vi "sine_plotter.vi"() -> ()   [LabVIEW 2014]
panel:
  out "XY Graph":cluster{"XArray":dbl[], "YArray":dbl[]}(graph)
  out "YArray":dbl[](array[numeric])
  out "XArray":dbl[](array[numeric])
  out "XSteps":dbl
  in  "XEnd":dbl
  in  "XRes":dbl
  in  "XStart":dbl
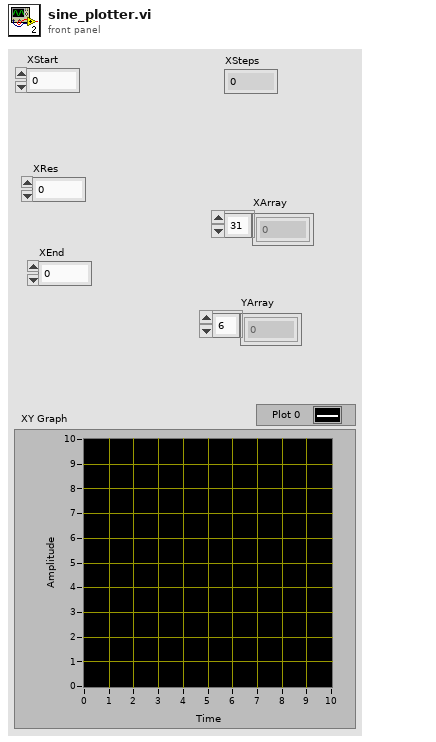
[diagram p1: front panel]
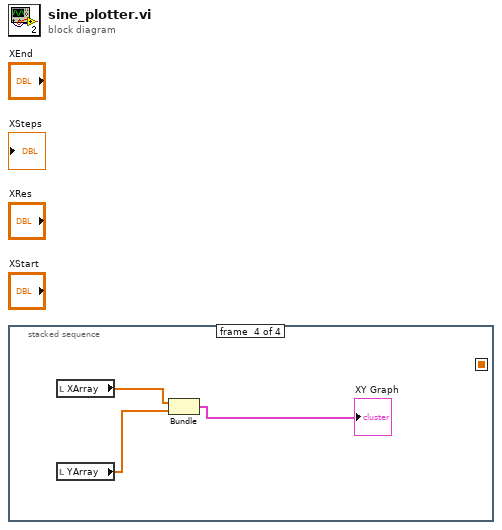
[diagram p0: block diagram]
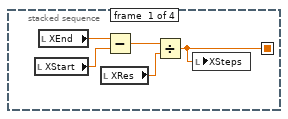
[diagram p2: hidden frame]
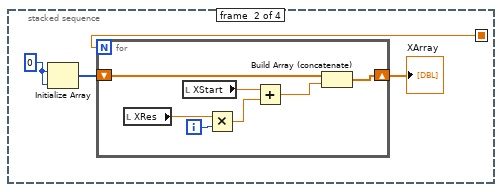
[diagram p3: hidden frame]
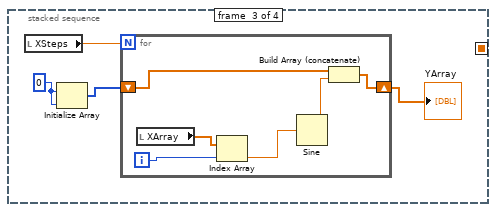
[diagram p4: hidden frame]
diagram:
  n1 = stacked-sequence {
    seq-local: [w1 _ _ _] -> [_ w9 _ _]
    frame #0 {
      n2 = local read "XStart"() -> (w4:dbl)
      n3 = local read "XEnd"() -> (w5:dbl)
      n4 = local read "XRes"() -> (w2:dbl)
      n5 = Subtract(x=w5, y=w4) -> (x-y=w3:dbl)
      n6 = Divide(x=w3, y=w2) -> (x/y=w1:dbl)
      n7 = local write "XSteps"(w1) -> ()
    }
    frame #1 {
      w8 = 0
      n8 = Initialize Array(w8, w8) -> (w7:i32[])
      n9 = for {
        N: w9 -> [_]
        shift-right: [w10] -> w6
        shift-left: w7 -> [w12]
        i -> [w15]
        n10 = local read "XRes"() -> (w16:dbl)
        n11 = local read "XStart"() -> (w14:dbl)
        n12 = Multiply(x=w16, y=w15) -> (x*y=w13:dbl)
        n13 = Add(x=w14, y=w13) -> (x+y=w11:dbl)
        n14 = Build Array (concatenate)(w12, w11) -> (w10:dbl[])
      }
      "XArray" <- w6
    }
    frame #2 {
      w19 = 0
      n15 = local read "XSteps"() -> (w20:dbl)
      n16 = Initialize Array(w19, w19) -> (w18:i32[])
      n17 = for {
        N: w20 -> [_]
        shift-right: [w21] -> w17
        shift-left: w18 -> [w23]
        i -> [w26]
        n18 = local read "XArray"() -> (w25:dbl[])
        n19 = Index Array(array=w25, index=w26) -> (element=w24:dbl)
        n20 = Sine(x=w24) -> (sin(x)=w22:dbl)
        n21 = Build Array (concatenate)(w23, w22) -> (w21:dbl[])
      }
      "YArray" <- w17
    }
    frame #3 {
      n22 = local read "XArray"() -> (w29:dbl[])
      n23 = local read "YArray"() -> (w28:dbl[])
      n24 = Bundle("XArray"=w29, "YArray"=w28) -> (→"XY Graph":cluster{"XArray":dbl[], "YArray":dbl[]})  [unwired: 1 in]
    }
  }
